vi "DPC_Read_Data.vi"(8 "error in":errorcluster, 11 "VISA in":refnum<visa-resource-name>) -> (0 "error out":errorcluster, 2 "DataOut":u16[][](array[numeric]), 3 "VISA out":refnum<visa-resource-name>, 4 "Error":bool)   [LabVIEW 2019]
uses:
  SiPM_Tests_Global_Var.vi
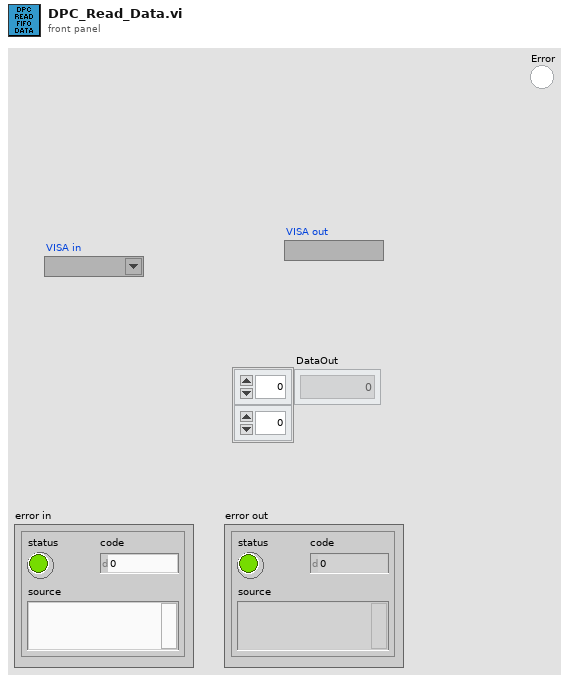
[diagram p1: front panel]
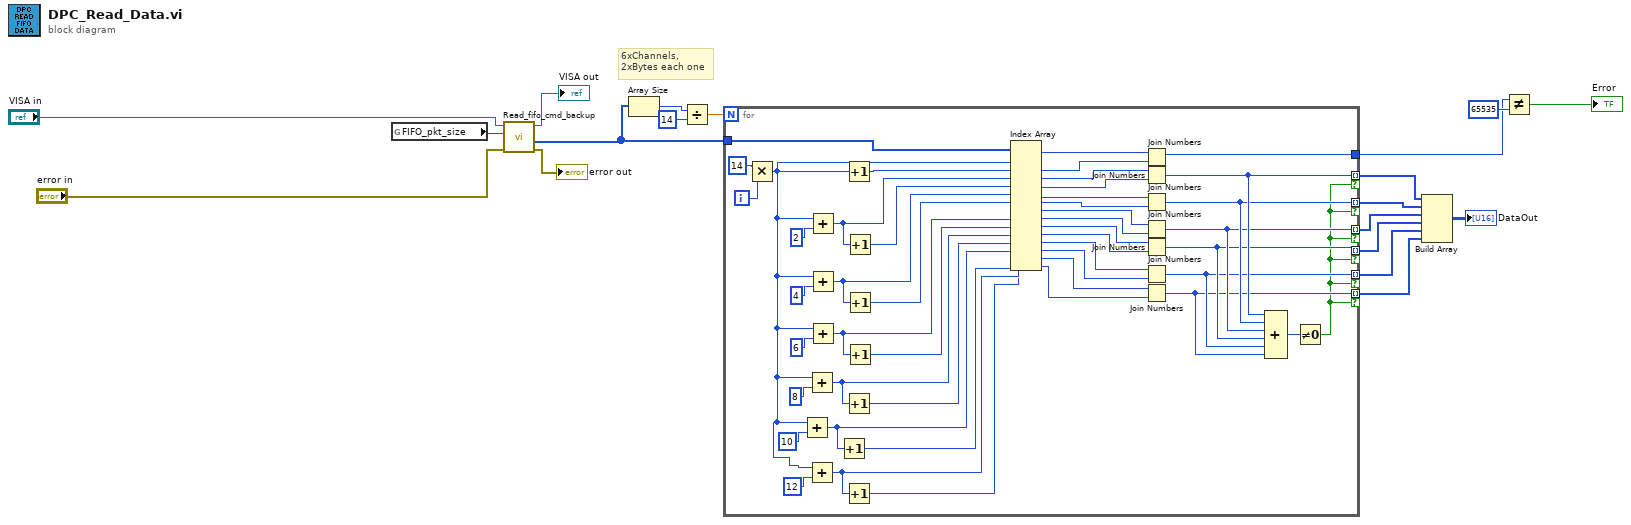
[diagram p0: block diagram]
diagram:
  # "6xChannels, \n2xBytes each one"
  n1 = global read "SiPM_Tests_Global_Var.vi" "FIFO_pkt_size"() -> (w12:u16)
  n2 = call "Read_fifo_cmd_backup.vi"("error in (no error)"="error in", "FIFO_pkt_size"=w12, "VISA Refnum in"="VISA in") -> ("error out"=→"error out":errorcluster, "Data_out"=w2:u8[], "VISA Refnum out"=→"VISA out":refnum<visa-resource-name>)  [unwired: 6 in]
  n3 = Array Size(array=w2) -> (size(s)=w15:i32)
  n4 = Divide(x=w15, y=u16 14) -> (x/y=w14:dbl)
  n5 = for {
    N: w14 -> [_]
    tunnel: w2 -> [w63]
    tunnel: [w62] -> w1
    tunnel: [w28] -> w11 mode=indexing if=w21
    tunnel: [w27] -> w10 mode=indexing if=w21
    tunnel: [w26] -> w9 mode=indexing if=w21
    tunnel: [w25] -> w8 mode=indexing if=w21
    tunnel: [w24] -> w7 mode=indexing if=w21
    tunnel: [w23] -> w3 mode=indexing if=w21
    i -> [w65]
    n6 = Multiply(x=14, y=w65) -> (x*y=w33:i32)
    n7 = Add(x=w33, y=10) -> (x+y=w38:i32)
    n8 = Add(x=w33, y=8) -> (x+y=w42:i32)
    n9 = Add(x=w33, y=12) -> (x+y=w32:i32)
    n10 = Add(x=w33, y=2) -> (x+y=w59:i32)
    n11 = Add(x=w33, y=4) -> (x+y=w56:i32)
    n12 = Add(x=w33, y=6) -> (x+y=w53:i32)
    n13 = Increment(x=w38) -> (x+1=w39:i32)
    n14 = Increment(x=w33) -> (x+1=w61:i32)
    n15 = Increment(x=w42) -> (x+1=w41:i32)
    n16 = Increment(x=w32) -> (x+1=w31:i32)
    n17 = Increment(x=w59) -> (x+1=w58:i32)
    n18 = Increment(x=w56) -> (x+1=w55:i32)
    n19 = Increment(x=w53) -> (x+1=w52:i32)
    n20 = Index Array(array=w63, index #1=w33, index #2=w61, index #3=w59, index #4=w58, index #5=w56, index #6=w55, index #7=w53, index #8=w52, index #9=w42, index #10=w41, index #11=w38, index #12=w39, index #13=w32, index #14=w31) -> (element #1=w51:u8, element #2=w50:u8, element #3=w49:u8, element #4=w48:u8, element #5=w47:u8, element #6=w46:u8, element #7=w45:u8, element #8=w44:u8, element #9=w20:u8, element #10=w37:u8, element #11=w36:u8, element #12=w35:u8, element #13=w30:u8, element #14=w29:u8)
    n21 = Join Numbers(hi=w51, lo=w50) -> ((hi.lo)=w62:u16)
    n22 = Join Numbers(hi=w49, lo=w48) -> ((hi.lo)=w28:u16)
    n23 = Join Numbers(hi=w47, lo=w46) -> ((hi.lo)=w27:u16)
    n24 = Join Numbers(hi=w45, lo=w44) -> ((hi.lo)=w26:u16)
    n25 = Join Numbers(hi=w20, lo=w37) -> ((hi.lo)=w25:u16)
    n26 = Join Numbers(hi=w36, lo=w35) -> ((hi.lo)=w24:u16)
    n27 = Join Numbers(hi=w30, lo=w29) -> ((hi.lo)=w23:u16)
    n28 = Compound Arithmetic op=ADD(w28, w27, w26, w25, w24, w23) -> (w22:u16)
    n29 = Not Equal To 0?(x=w22) -> (x != 0?=w21:bool)
  }
  n30 = Build Array(w11, w10, w9, w8, w7, w3) -> (→"DataOut":u16[][])
  n31 = Not Equal?(x=w1, y=u16 65535) -> (x != y?=→"Error":bool)
